vi "Modify Current SN.vi"(8 "error in (no error)":errorcluster) -> (0 "error out":errorcluster)   [LabVIEW 2017]
uses:
  <vilib>/Utility/config.llb/Read Key (U32).vi
  <vilib>/Utility/config.llb/Read Key (String).vi
  <vilib>/Utility/config.llb/Write Key (U32).vi
  <vilib>/Utility/config.llb/Write Key (String).vi
  <vilib>/Utility/config.llb/NI_LVConfig.lvlib
panel:
  out "Date":string
  in  "SERIAL NUMBER":u32=1 min=1 max=999999 step=1
  in  "SAVE":bool
  in  "stop":bool
  in  "PART CODE":string(combo)
  # "MODIFY CURRENT SN"
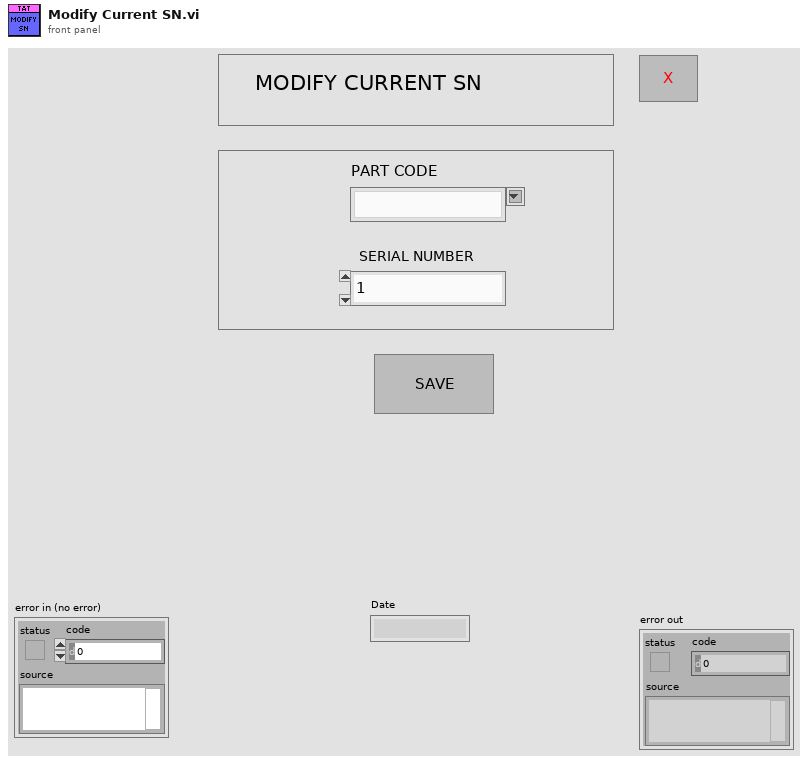
[diagram p1: front panel]
types:
  T1 = enum32{"invalid app kind", "Development System", "Run Time System", "Student Edition", "Embedded LabVIEW", "Evaluation", "Custom"}
  T2 = typedef "NI_LVConfig.lvlib/Config Data RefNum.ctl" = refnum<k1>
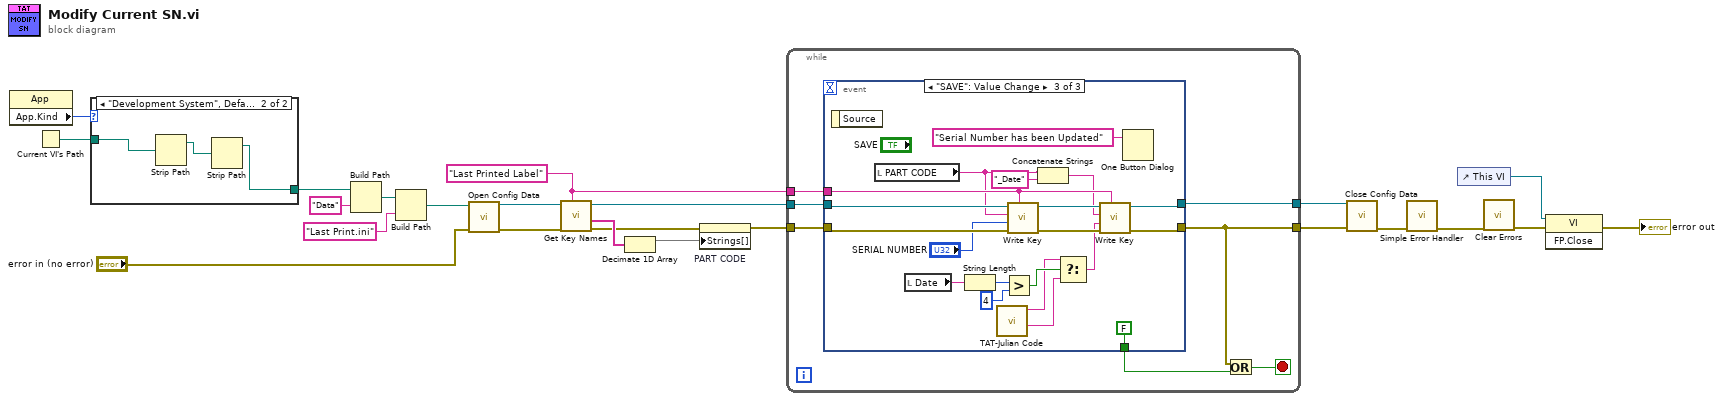
[diagram p0: block diagram]
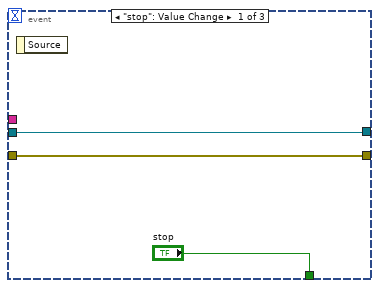
[diagram p2: hidden frame]
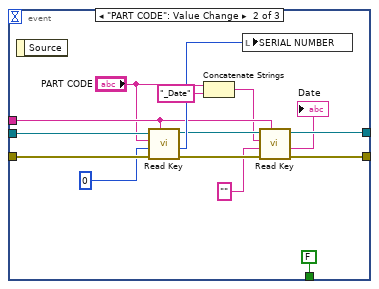
[diagram p3: hidden frame]
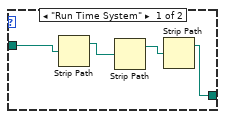
[diagram p4: hidden frame]
diagram:
  w6 = "Last Printed Label" ("section")
  n1 = property class="App"() -> ("App.Kind"=w22:T1)  [unwired: 2 in, 2 out]
  n2 = Current VI's Path() -> (path=w23:path)
  n3 = case shown="\"Development System\", Default" w22 {
    tunnel: w23 -> [w25 w29]
    tunnel: [w24 w28] -> w20
    frame "Run Time System" {
      n4 = Strip Path(path=w25) -> (stripped path=w27:path)  [unwired: 1 out]
      n5 = Strip Path(path=w27) -> (stripped path=w26:path)  [unwired: 1 out]
      n6 = Strip Path(path=w26) -> (stripped path=w24:path)  [unwired: 1 out]
    }
    frame "Development System", Default {
      n7 = Strip Path(path=w29) -> (stripped path=w30:path)  [unwired: 1 out]
      n8 = Strip Path(path=w30) -> (stripped path=w28:path)  [unwired: 1 out]
    }
  }
  n9 = Build Path(base path=w20, name or relative path="Data") -> (appended path=w19:path)
  n10 = Build Path(base path=w19, name or relative path="Last Print.ini") -> (appended path=w17:path)
  n11 = call <vilib>:"Open Config Data.vi"("error in (no error)"="error in (no error)", "configuration file path"=w17) -> ("error out"=w14:errorcluster, "refnum"=w16:T2)  [unwired: 7 in, 1 out]
  n12 = call <vilib>:"Get Key Names.vi"("section"=w6, "error in (no error)"=w14, "refnum"=w16) -> ("error out"=w11:errorcluster, "key names"=w13:string[], "refnum out"=w8:T2)  [unwired: 5 in, 1 out]
  n13 = Decimate 1D Array(w13) -> (w12:string[])  [unwired: 1 out]
  n14 = property on="PART CODE" class="CmbBox"(error in=w11, "Strings[]"=w12) -> (error out=w10:errorcluster)  [unwired: 1 in, 1 out]
  n15 = while {
    tunnel: w10 -> [w36]
    tunnel: [w31] -> w9
    tunnel: w8 -> [w35]
    tunnel: [w34] -> w7
    tunnel: w6 -> [w33]
    stop <- w32 stop-if-true
    n16 = event shown="[2] \"SAVE\": Value Change" {
      selector: _ -> [_ _ _]
      dyn-events: _ -> [_ _ _]
      timeout: _ -> [_ _ _]
      tunnel: ["stop" FALSE ("stop") FALSE ("stop")] -> w37
      tunnel: w36 -> [w38 w54 w75]
      tunnel: [w38 w47 w67] -> w31
      tunnel: w35 -> [w39 w53 w74]
      tunnel: [w39 w49 w69] -> w34
      tunnel: w33 -> [_ w46 w66]
      event "stop": Value Change {
        n17 = event-data() -> ()  [unwired: 1 in, 1 out]
      }
      event "PART CODE": Value Change {
        n18 = event-data() -> ()  [unwired: 1 in, 1 out]
        n19 = call-poly <vilib>:"Read Key.vi"("section"=w46, "error in (no error)"=w54, "default value"=u32 0, "key"="PART CODE", "refnum"=w53) -> ("error out"=w48:errorcluster, "value"=w51:u32, "refnum out"=w50:T2)  [unwired: 3 in, 1 out]
        n20 = Concatenate Strings("PART CODE", "_Date" ("string")) -> (w43:string)
        n21 = local write "SERIAL NUMBER"(w51) -> ()
        n22 = call-poly <vilib>:"Read Key.vi"("section"=w46, "error in (no error)"=w48, "default value"="", "key"=w43, "refnum"=w50) -> ("error out"=w47:errorcluster, "value"=→"Date":string, "refnum out"=w49:T2)  [unwired: 3 in, 1 out]
      }
      event "SAVE": Value Change {
        n23 = event-data() -> ()  [unwired: 1 in, 1 out]
        n24 = local read "PART CODE"() -> (w65:string)
        n25 = local read "Date"() -> (w61:string)
        n26 = String Length(string=w61) -> (length=w60:i32)
        n27 = call "TAT-Julian Code.vi"() -> ("Short Date"=w56:string, "Julian Code"=w57:string)  [unwired: 8 in, 2 out]
        n28 = Greater?(x=w60, y=4) -> (0:w58:bool)
        n29 = call-poly <vilib>:"Write Key.vi"("section"=w66, "error in (no error)"=w75, "value"="SERIAL NUMBER", "key"=w65, "refnum"=w74) -> ("error out"=w68:errorcluster, "refnum out"=w70:T2)  [unwired: 4 in, 1 out]
        n30 = Concatenate Strings(w65, "_Date" ("string")) -> (w63:string)
        n31 = Select(t=w57, s=w58, f=w56) -> (s? t:f=w62:string)
        n32 = call-poly <vilib>:"Write Key.vi"("section"=w66, "error in (no error)"=w68, "value"=w62, "key"=w63, "refnum"=w70) -> ("error out"=w67:errorcluster, "refnum out"=w69:T2)  [unwired: 4 in, 1 out]
        n33 = One Button Dialog(message="Serial Number has been Updated") -> ()  [unwired: 1 in, 1 out]
      }
    }
    n34 = Or(x=w31, y=w37) -> (x .or. y?=w32:bool)
  }
  n35 = call <vilib>:"Close Config Data.vi"("error in (no error)"=w9, "refnum"=w7) -> ("error out"=w5:errorcluster)  [unwired: 8 in, 1 out]
  n36 = call <vilib>:"Simple Error Handler.vi"("error in (no error)"=w5) -> ("error out"=w4:errorcluster)  [unwired: 4 in, 4 out]
  n37 = control-ref of="This VI"() -> (w1:refnum<vi>)
  n38 = call <vilib>:"Clear Errors.vi"("error in (no error)"=w4) -> ("error out"=w3:errorcluster)  [unwired: 5 in, 1 out]
  n39 = invoke class="VI" method="FP.Close"(reference=w1, error in=w3) -> (error out=→"error out":errorcluster)  [unwired: 1 in, 2 out]
